vi "valve_Z_state init.vi"(10 "N_param":i32) -> (0 "error":errorcluster, 3 "Z_states":T1)   [LabVIEW 2019, in "Valves.lvlib"]
uses:
  Valves.lvlib
  Inputs/Ctl/AI scada.ctl
  Inputs/Inputs.lvlib
  Heating/ctl/Z_source.ctl
  Heating/Heating.lvlib
  ctl/Z_State_VCH.ctl
  ctl/ZM_State_VCH.ctl
  ctl/Z.ctl
panel:
  # "Analog parameters"
  # "Description of analog parameters"
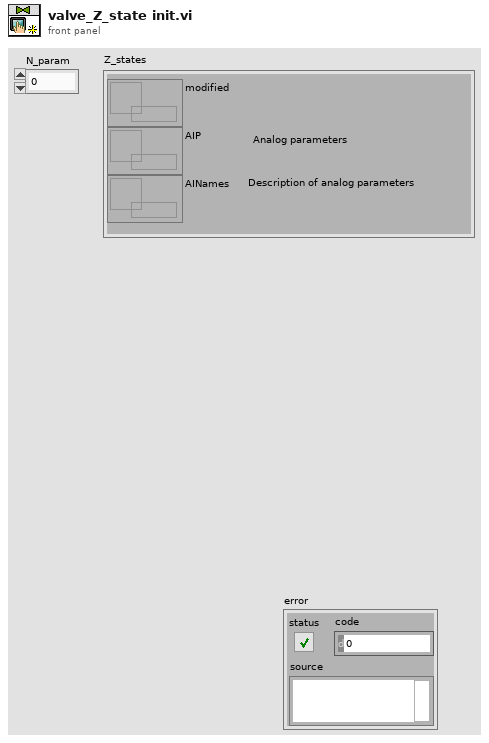
[diagram p1: front panel]
types:
  T1 = typedef "Inputs.lvlib/AI scada.ctl" = cluster{"modified":refnum<data-value>, "AIP":refnum<data-value>, "AINames":refnum<data-value>}
  T2 = typedef "Valves.lvlib/Z.ctl" = cluster{"Z_Source":T3, "Z_SetState":T4, "Z_State":T4, "Z_State_T":u32, "ZM_State":T5, "ZM_State_T":u32, "ALR  L1":bool, "ALR  L2":bool, "HH_run":i32}
  T3 = typedef "Heating.lvlib/Z_source.ctl" = enum8{"initialize", "local disabled", "local hand", "hand", "auto", "dist"}
  T4 = typedef "Valves.lvlib/Z_State_VCH.ctl" = enum8{"initialization", "alarm", "disabled", "not ready", "closed ready", "reserv", "reserv1", "reserv2", "reserv3", "check", "on min", "open", "on (closed)"}
  T5 = typedef "Valves.lvlib/ZM_State_VCH.ctl" = enum8{"initialization", "closed", "big_pause", "little_pause", "open", "close_cmd"}
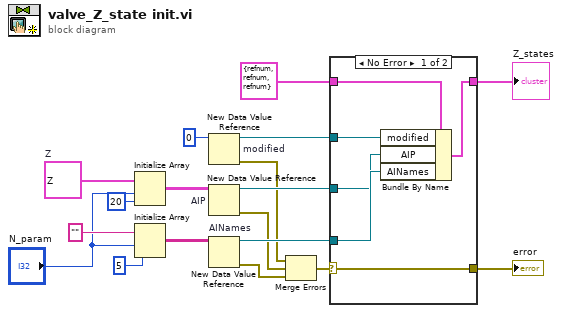
[diagram p0: block diagram]
diagram:
  w1 = T2 {"Z_Source"=enum."local disabled", "Z_SetState"=enum."initialization", "Z_State"=enum."initialization", "Z_State_T"=0, "ZM_State"=enum."initialization", "ZM_State_T"=0, "ALR  L1"=FALSE, "ALR  L2"=FALSE, "HH_run"=0}  # Z
  n1 = Initialize Array(w1, "N_param", 20 ("dimension size")) -> (w8:T2[][])
  n2 = Initialize Array("" ("AINames"), "N_param", 5 ("dimension size")) -> (w15:string[][])
  n3 = New Data Value Reference "modified"(data value=u8 0 ("modified")) -> (data value reference=w3:refnum<data-value>, error out=w4:errorcluster)  [unwired: 1 in]
  n4 = New Data Value Reference "AIP"(data value=w8) -> (data value reference=w7:refnum<data-value>, error out=w5:errorcluster)  [unwired: 1 in]
  n5 = New Data Value Reference "AINames"(data value=w15) -> (data value reference=w14:refnum<data-value>, error out=w9:errorcluster)  [unwired: 1 in]
  n6 = Merge Errors(w4, w5, w9) -> (w6:errorcluster)
  n7 = case shown="No Error" w6 {
    selector: w6 -> [w22 w26]
    tunnel: w7 -> [w20 _]
    tunnel: w14 -> [w21 _]
    tunnel: [w22 w26] -> w12
    tunnel: T1 {"modified"=refnum, "AIP"=refnum, "AINames"=refnum} ("AI") -> [w24 w25]
    tunnel: [w23 w25] -> w10
    tunnel: w3 -> [w19 _]
    frame No Error {
      n8 = Bundle By Name(cluster=w24, "modified"=w19, "AIP"=w20, "AINames"=w21) -> (w23:T1)
    }
    frame Error {
    }
  }
  "error" <- w12
  "Z_states" <- w10
